vi "Scale Frequency.vi"(1 "Period":dbl[unit]) -> (0 "Frequency (scaled)":u32)   [LabVIEW 2009]
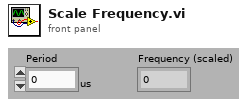
[diagram p1: front panel]
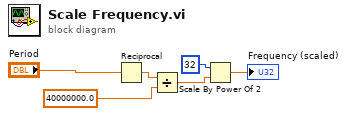
[diagram p0: block diagram]
diagram:
  n1 = Reciprocal(x="Period") -> (1/x=w4:dbl[unit])
  n2 = Divide(x=w4, y=dbl[unit] 40000000.0) -> (x/y=w6:dbl)
  n3 = Scale By Power Of 2(n=i16 32, x=w6) -> (x*2^n=→"Frequency (scaled)":dbl)
